vi "MessageName.vi"() -> (2 "MessageName":string)   [LabVIEW 2023, in "ConstellationCommand.lvlib"]
uses:
  ConstellationCommand.lvlib
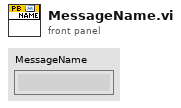
[diagram p1: front panel]
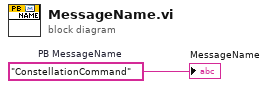
[diagram p0: block diagram]
diagram:
  w1 = "ConstellationCommand"  # PB MessageName
  "MessageName" <- w1
